vi "AlliGator Get-Set Phasor Plot Reference is Updated.vi"(6 "Set/Get (F)":bool, 8 "error in (no error)":errorcluster, 11 "Phasor Plot Reference Updated":bool) -> (0 "error out":errorcluster, 3 "Phasor Plot Reference Updated ?":bool)   [LabVIEW 2021, in "AlliGator Phasor Plot.lvlib"]
doc: "Stores status of Phasor Plot references changes."
uses:
  AlliGator Phasor Plot.lvlib
panel:
  # "see the AlliGator License on the block diagram (Ctrl+E or Window:Show Block Diagram)"
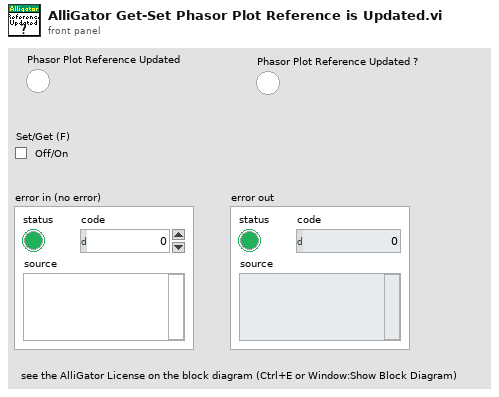
[diagram p1: front panel]
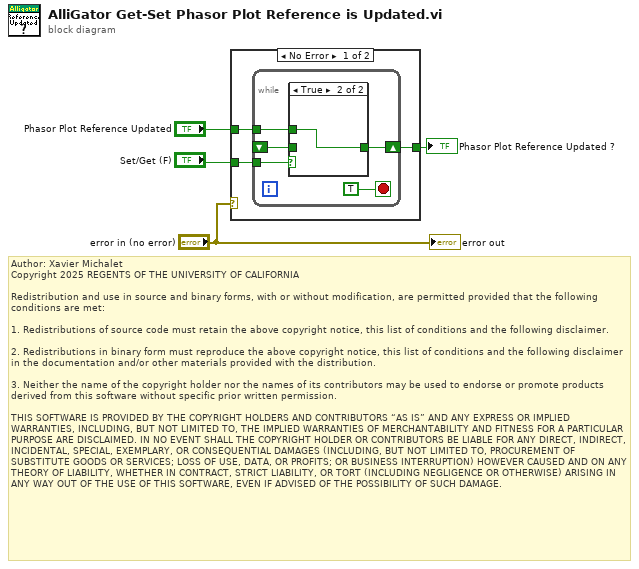
[diagram p0: block diagram]
diagram:
  # "Author: Xavier Michalet\nCopyright 2025 REGENTS OF THE UNIVERSITY OF CALIFORNIA\n\nRedistribution and use in source and binary forms, with or without modification, are permitted provided that the following conditions are met:\n\n1. Redistributions of source code must retain the above copyright notice, this list of conditions and the following disclaimer.\n\n2. Redistributions in binary form must reproduce the above copyright notice, this list of conditions and the following disclaimer in the documentation and/or other materials provided with the distribution.\n\n3. Neither the name of the copyright holder nor the names of its contributors may be used to endorse or promote products derived from this software without specific prior written permission.\n\nTHIS SOFTWARE IS PROVIDED BY THE COPYRIGHT HOLDERS AND CONTRIBUTORS “AS IS” AND ANY EXPRESS OR IMPLIED WARRANTIES, INCLUDING, BUT NOT LIMITED TO, THE IMPLIED WARRANTIES OF MERCHANTABILITY AND FITNESS FOR A PARTICULAR PURPOSE ARE DISCLAIMED. IN NO EVENT SHALL THE COPYRIGHT HOLDER OR CONTRIBUTORS BE LIABLE FOR ANY DIRECT, INDIRECT, INCIDENTAL, SPECIAL, EXEMPLARY, OR CONSEQUENTIAL DAMAGES (INCLUDING, BUT NOT LIMITED TO, PROCUREMENT OF SUBSTITUTE GOODS OR SERVICES; LOSS OF USE, DATA, OR PROFITS; OR BUSINESS INTERRUPTION) HOWEVER CAUSED AND ON ANY THEORY OF LIABILITY, WHETHER IN CONTRACT, STRICT LIABILITY, OR TORT (INCLUDING NEGLIGENCE OR OTHERWISE) ARISING IN ANY WAY OUT OF THE USE OF THIS SOFTWARE, EVEN IF ADVISED OF THE POSSIBILITY OF SUCH DAMAGE."
  n1 = case shown="No Error" "error in (no error)" {
    tunnel: "Set/Get (F)" -> [w7 _]
    tunnel: "Phasor Plot Reference Updated" -> [w6 w15]
    tunnel: [w5 w15] -> w2
    frame No Error {
      n2 = while {
        tunnel: w7 -> [w11]
        tunnel: w6 -> [w10]
        shift-right: [w9] -> w5
        shift-left: _ -> [w8]
        stop <- TRUE stop-if-true
        n3 = case shown="True" w11 {
          tunnel: w10 -> [_ w14]
          tunnel: [w13 w14] -> w9
          tunnel: w8 -> [w13 _]
          frame False {
          }
          frame True {
          }
        }
      }
    }
    frame Error {
    }
  }
  "Phasor Plot Reference Updated ?" <- w2
  "error out" <- "error in (no error)"
